vi "PowderDeposition.vi"(8 "error in (no error)":errorcluster, 9 "Com-in":refnum<queue>, 10 "Com-out":refnum<queue>) -> (0 "error out":errorcluster)   [LabVIEW 2013, in "PowderDeposition.lvlib"]
doc: "Use this template to build a producer/consumer design pattern with events to produce queue items. Use this design pattern instead of the User Interface Event Handler pattern for user interfaces when you want to execute code asynchronously in response to an event without slowing the user interface responsiveness."
uses:
  PowderDeposition.lvlib
  Sources/Assembly/Motor-selection.ctl
  Sources/Action/Motor-actions.ctl
  Sources/Main/Options.ctl
  SA-SLMAPI/Sources/Message.lvclass
  Sources/Main/Motor-status.ctl
  Sources/Main/PD-actions.ctl
  Sources/Main/Enqueue-modes.ctl
  Sources/Main/Client-status.ctl
  Sources/Main/Execution-actions.ctl
  Sources/Main/PD-Main.lvclass/PD-Main.ctl
  Sources/Main/Read Assert safe.vi
  Sources/Main/PD-Main.lvclass
  Sources/Assembly/Motor-assembly.lvclass
  Sources/Action/Action.lvclass
panel:
  in  "Clear sequences":bool
  in  "Save sequences":bool
  in  "Load sequences":bool
  in  "Edit action":bool
  in  "Remove from sequence":bool
  in  "Add to sequence":bool
  in  "Available-actions":T1=enum."Move - Relative" caption="Action"
  in  "Execute sequence":bool
  in  "Execute action":bool
  in  "Quick stop":bool
  in  "Toggle help":bool
  out "Motors-status":T2 caption="Status"
  in  "Options":T3
  in  "Activate all":bool
  in  "De-activate all":bool
  in  "Motors-selection":T4 caption="Select motors"
  in  "Motor tabs":T5(tab)
  in  "M1-sequence":i32(listbox) caption="M1 - Action sequence"
  in  "M2-sequence":i32(listbox) caption="M2 - Action sequence"
  in  "M3-sequence":i32(listbox) caption="M3 - Action sequence"
  in  "M4-sequence":i32(listbox) caption="M4 - Action sequence"
  out "Log":string[][](table)
  out "Status":string caption="Status:"
  out "Action:":T6
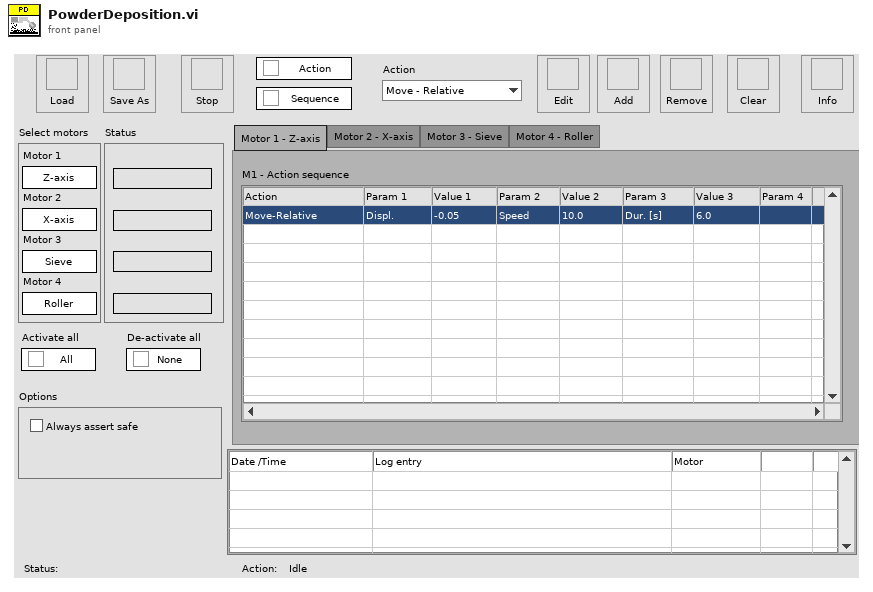
[diagram p1: front panel]
types:
  T1 = typedef "PowderDeposition.lvlib/Action.lvclass/Motor-actions.ctl" = enum16{"Move - Absolute", "Move - Relative", "Move - Timer", "Wait", "Home", "Substrate", "Sieve", "Stop"}
  T2 = typedef "PowderDeposition.lvlib/PD-Main.lvclass/Motor-status.ctl" = cluster{"Motor 1 status":string, "Motor 2 status":string, "Motor 3 status":string, "Motor 4 status":string}
  T3 = typedef "PowderDeposition.lvlib/PD-Main.lvclass/Options.ctl" = cluster{"Assert safe":bool}
  T4 = typedef "PowderDeposition.lvlib/Motor-assembly.lvclass/Motor-selection.ctl" = cluster{"Motor 1":bool, "Motor 2":bool, "Motor 3":bool, "Motor 4":bool}
  T5 = enum32{"Motor 1 - Z-axis", "Motor 2 - X-axis", "Motor 3 - Sieve", "Motor 4 - Roller"}
  T6 = typedef "PowderDeposition.lvlib/PD-Main.lvclass/PD-actions.ctl" = enum16{"Idle", "Initialize", "Signal initialized", "Activate all motors", "Deactivate all motors", "Update motor activity", "Update selected motor", "Update motor status", "Update selected sequence", "Load sequences with dialog", "Load sequences from file", "Save sequences", "Add to sequence", "Remove from sequence", "Clear sequences", "Update available actions", "Create action", "Edit action", "Execute action", "Execute sequences", "Execute seq with assert", "Abort", "Exit"}
  T7 = typedef "PowderDeposition.lvlib/PD-Main.lvclass/Object-reference.ctl" = refnum<data-value>
  T8 = typedef "PowderDeposition.lvlib/PD-Main.lvclass/Client-status.ctl" = enum16{"Idle", "Initialized", "Configured", "Activated", "Started", "Paused", "Stopped", "Reset", "Error", "Exited"}
  T9 = typedef "PowderDeposition.lvlib/PD-Main.lvclass/Execution-actions.ctl" = enum16{"Idle", "Execute action", "Execute sequence", "Execute seq with assert", "Exit"}
  T10 = typedef "PowderDeposition.lvlib/PD-Main.lvclass/Enqueue-modes.ctl" = enum16{"Default", "Priority", "Flush"}
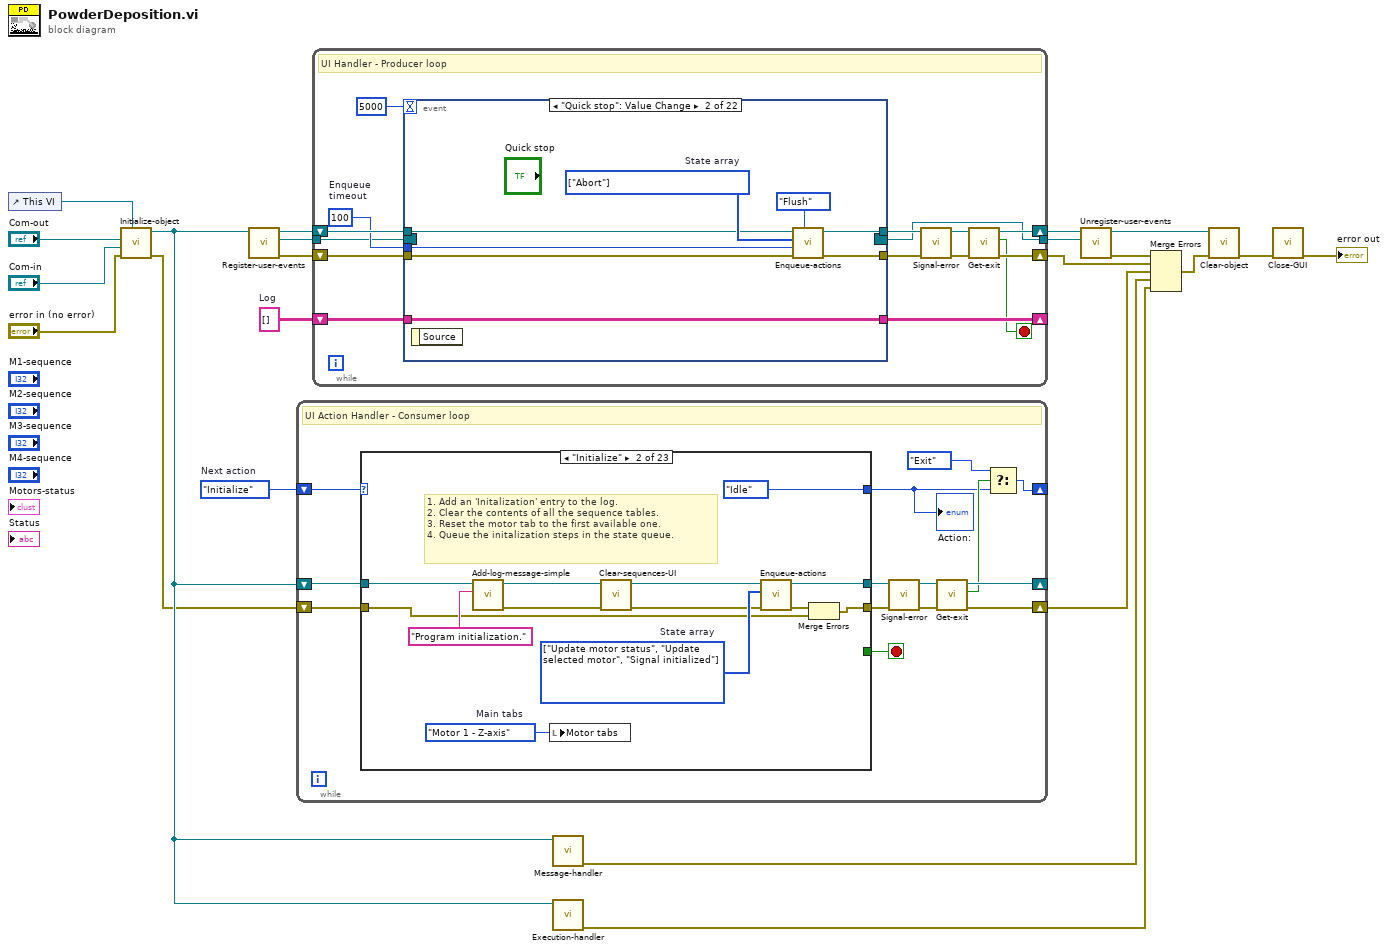
[diagram p0: block diagram]
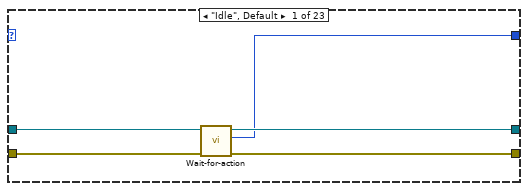
[diagram p2: hidden frame]
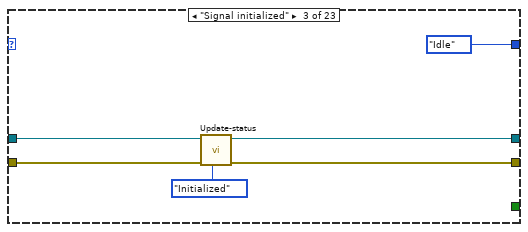
[diagram p3: hidden frame]
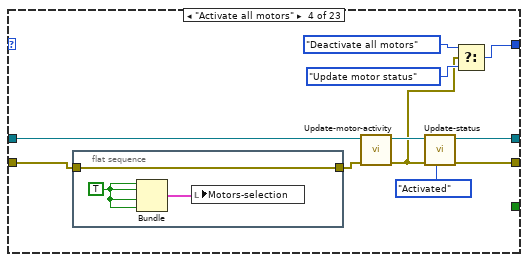
[diagram p4: hidden frame]
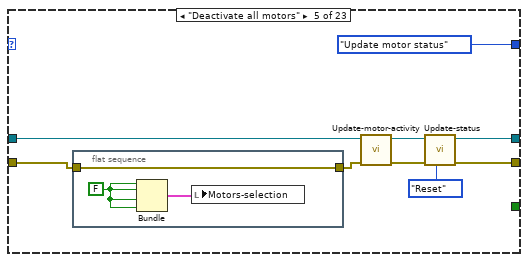
[diagram p5: hidden frame]
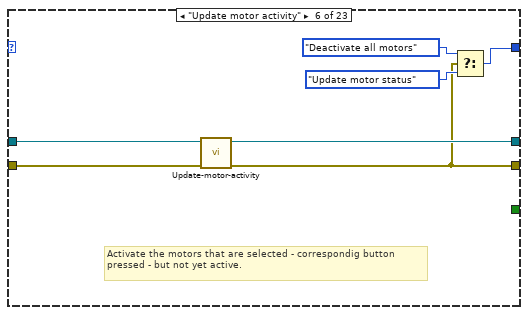
[diagram p6: hidden frame]
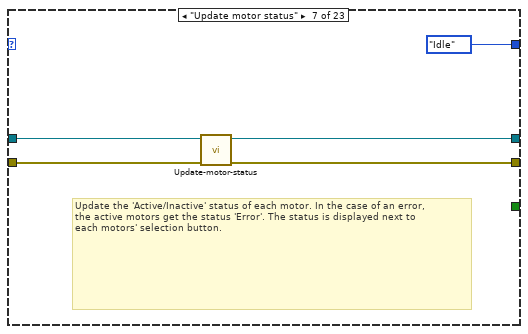
[diagram p7: hidden frame]
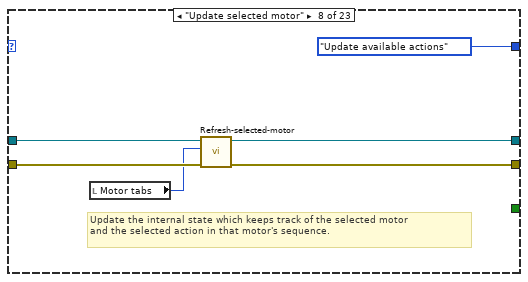
[diagram p8: hidden frame]
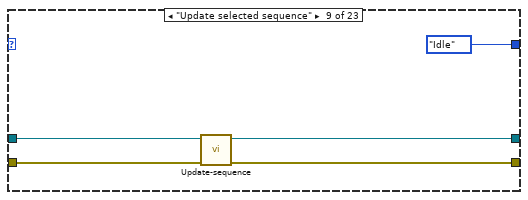
[diagram p9: hidden frame]
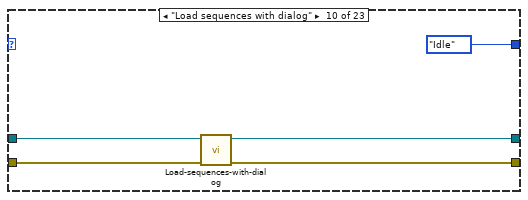
[diagram p10: hidden frame]
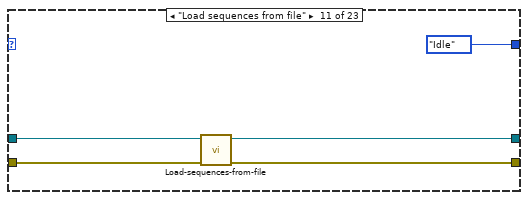
[diagram p11: hidden frame]
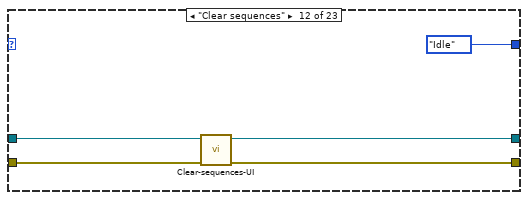
[diagram p12: hidden frame]
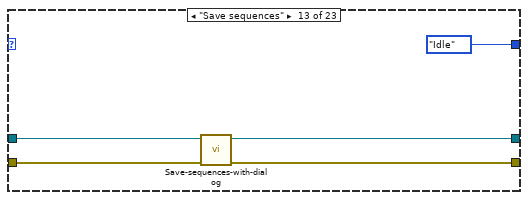
[diagram p13: hidden frame]
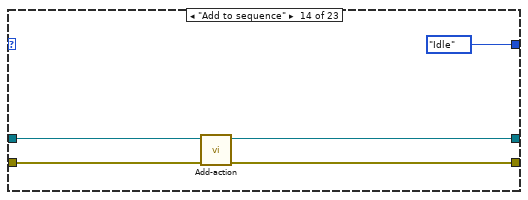
[diagram p14: hidden frame]
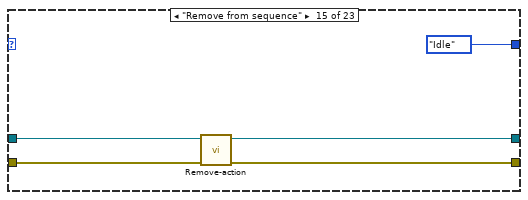
[diagram p15: hidden frame]
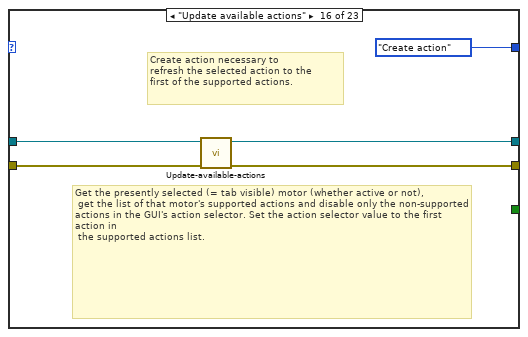
[diagram p16: hidden frame]
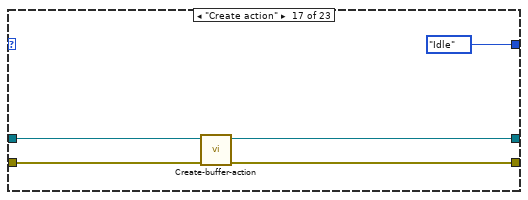
[diagram p17: hidden frame]
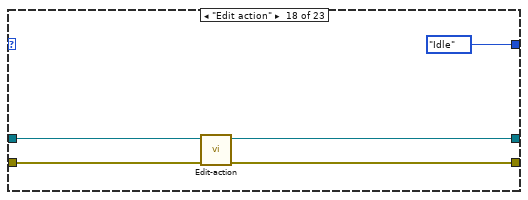
[diagram p18: hidden frame]
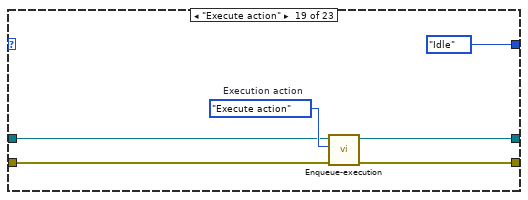
[diagram p19: hidden frame]
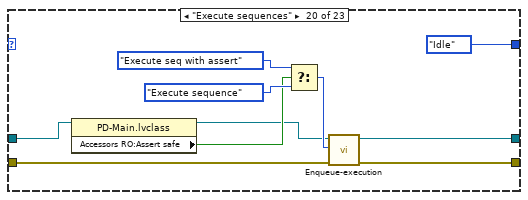
[diagram p20: hidden frame]
diagram:
  w20 = string[][] []  # Log
  w22 = PD-actions."Initialize"  # Next action
  n1 = control-ref of="This VI"() -> (w17:refnum<vi>)
  n2 = call "Initialize-object.vi"("Main VI ref"=w17, "error in (no error)"="error in (no error)", "Client channel"="Com-in", "Server channel"="Com-out") -> ("error out"=w4:errorcluster, "Object ref out"=w7:T7)  [unwired: 6 in]
  n3 = call "Register-user-events.vi"("Object ref in"=w7) -> ("error out"=w14:errorcluster, "Event registration"=w15:refnum<event-registration>, "Object ref out"=w16:T7)  [unwired: 8 in]
  n4 = while {
    shift-right: [w27] -> _
    shift-left: w22 -> [w35]
    shift-right: [w25] -> w21
    shift-left: w4 -> [w34]
    shift-right: [w30] -> _
    shift-left: w7 -> [w33]
    stop <- w36 stop-if-true
    # "UI Action Handler - Consumer loop"
    n5 = case shown="\"Initialize\"" w35 {
      tunnel: [_ _ _ _ _ _ _ _ _ _ _ _ _ _ _ _ _ _ _ _ _ _ TRUE] -> w36
      tunnel: w34 -> [w37 w44 w57 w69 w80 w92 w96 w100 w107 w112 w117 w122 w127 w132 w137 w143 w148 w152 w157 w161 w173 w179 w184]
      tunnel: [w39 w42 w56 w66 w76 w87 w95 w101 w105 w110 w115 w120 w125 w131 w135 w142 w145 w151 w156 w166 w175 w177 w187] -> w24
      tunnel: [w38 PD-actions."Idle" ("Action Handler states") PD-actions."Idle" ("Action Handler states") w62 PD-actions."Update motor status" ("Action Handler states") w88 PD-actions."Idle" ("Action Handler states") PD-actions."Update available actions" ("Action Handler states") PD-actions."Idle" ("Action Handler states") PD-actions."Idle" ("Action Handler states") PD-actions."Idle" ("Action Handler states") PD-actions."Idle" ("Action Handler states") PD-actions."Idle" ("Action Handler states") PD-actions."Idle" ("Action Handler states") PD-actions."Idle" ("Action Handler states") PD-actions."Create action" ("Action Handler states") PD-actions."Idle" ("Action Handler states") PD-actions."Idle" ("Action Handler states") PD-actions."Idle" ("Action Handler states") PD-actions."Idle" ("Action Handler states") PD-actions."Idle" ("Action Handler states") PD-actions."Idle" ("Action Handler states") PD-actions."Exit" ("Action Handler states")] -> w23
      tunnel: w33 -> [w41 w45 w58 w71 w82 w93 w97 w103 w108 w113 w118 w123 w128 w133 w138 w141 w147 w153 w158 w165 w172 w180 w186]
      tunnel: [w40 w51 w55 w65 w77 w91 w94 w102 w106 w111 w116 w121 w126 w130 w136 w140 w146 w150 w155 w163 w174 w178 w188] -> w32
      frame "Idle", Default {
        n6 = call "Wait-for-action.vi"("error in (no error)"=w37, "Object ref in"=w41) -> ("error out"=w39:errorcluster, "Next action"=w38:T6, "Object ref out"=w40:T7)  [unwired: 7 in]
      }
      frame "Initialize" {
        w48 = T5."Motor 1 - Z-axis"  # Main tabs
        w54 = T6[] [enum."Update motor status", enum."Update selected motor", enum."Signal initialized"] items=["Idle", "Initialize", "Signal initialized", "Activate all motors", "Deactivate all motors", "Update motor activity", "Update selected motor", "Update motor status", "Update selected sequence", "Load sequences with dialog", "Load sequences from file", "Save sequences", "Add to sequence", "Remove from sequence", "Clear sequences", "Update available actions", "Create action", "Edit action", "Execute action", "Execute sequences", "Execute seq with assert", "Abort", "Exit"]  # State array
        # "1. Add an 'Initalization' entry to the log.\n2. Clear the contents of all the sequence tables.\n3. Reset the motor tab to the first available one.\n4. Queue the initalization steps in the state queue."
        n7 = call "Add-log-message-simple.vi"("Message"="Program initialization." ("Log message"), "UI in"=w45) -> ("error out"=w49:errorcluster, "UI out"=w50:T7)  [unwired: 8 in]
        n8 = local write "Motor tabs"(w48) -> ()
        n9 = call "Clear-sequences-UI.vi"("error in (no error)"=w49, "Object ref in"=w50) -> ("error out"=w47:errorcluster, "Object ref out"=w46:T7)  [unwired: 8 in]
        n10 = call "Enqueue-actions.vi"("error in (no error)"=w47, "State array"=w54, "State queue in"=w46) -> ("error out"=w43:errorcluster, "State queue out"=w51:T7)  [unwired: 6 in, 1 out]
        n11 = Merge Errors(w43, w44) -> (w42:errorcluster)
      }
      frame "Signal initialized" {
        n12 = call "Update-status.vi"("Status"=Client-status."Initialized", "error in (no error)"=w57, "Object ref in"=w58) -> ("error out"=w56:errorcluster, "Object ref out"=w55:T7)  [unwired: 7 in]
      }
      frame "Activate all motors" {
        n13 = flat-sequence {
          tunnel: w69 -> [w72]
          tunnel: [w72] -> w70
          frame #0 {
            w73 = TRUE
            n14 = Bundle(w73, w73, w73, w73) -> (w74:cluster{bool, bool, bool, bool})  [unwired: 1 in]
            n15 = local write "Motors-selection"(w74) -> ()
          }
        }
        n16 = call "Update-motor-activity.vi"("error in (no error)"=w70, "Data in"=w71) -> ("error out"=w61:errorcluster, "Data out"=w67:T7)  [unwired: 8 in]
        n17 = call "Update-status.vi"("Status"=Client-status."Activated", "error in (no error)"=w61, "Object ref in"=w67) -> ("error out"=w66:errorcluster, "Object ref out"=w65:T7)  [unwired: 7 in]
        n18 = Select(t=PD-actions."Deactivate all motors" ("Action Handler states"), s=w61, f=PD-actions."Update motor status" ("Action Handler states")) -> (s? t:f=w62:T6)
      }
      frame "Deactivate all motors" {
        n19 = flat-sequence {
          tunnel: w80 -> [w84]
          tunnel: [w84] -> w81
          frame #0 {
            w85 = FALSE
            n20 = Bundle(w85, w85, w85, w85) -> (w86:cluster{bool, bool, bool, bool})  [unwired: 1 in]
            n21 = local write "Motors-selection"(w86) -> ()
          }
        }
        n22 = call "Update-motor-activity.vi"("error in (no error)"=w81, "Data in"=w82) -> ("error out"=w75:errorcluster, "Data out"=w78:T7)  [unwired: 8 in]
        n23 = call "Update-status.vi"("Status"=Client-status."Reset", "error in (no error)"=w75, "Object ref in"=w78) -> ("error out"=w76:errorcluster, "Object ref out"=w77:T7)  [unwired: 7 in]
      }
      frame "Update motor activity" {
        # "Activate the motors that are selected - correspondig button pressed - but not yet active."
        n24 = call "Update-motor-activity.vi"("error in (no error)"=w92, "Data in"=w93) -> ("error out"=w87:errorcluster, "Data out"=w91:T7)  [unwired: 8 in]
        n25 = Select(t=PD-actions."Deactivate all motors" ("Action Handler states"), s=w87, f=PD-actions."Update motor status" ("Action Handler states")) -> (s? t:f=w88:T6)
      }
      frame "Update motor status" {
        # "Update the 'Active/Inactive' status of each motor. In the case of an error,\nthe active motors get the status 'Error'. The status is displayed next to \neach motors' selection button."
        n26 = call "Update-motor-status.vi"("error in (no error)"=w96, "Object ref in"=w97) -> ("error out"=w95:errorcluster, "Object ref out"=w94:T7)  [unwired: 8 in]
      }
      frame "Update selected motor" {
        # "Update the internal state which keeps track of the selected motor\nand the selected action in that motor's sequence."
        n27 = local read "Motor tabs"() -> (w99:T5)
        n28 = call "Refresh-selected-motor.vi"("error in (no error)"=w100, "Motor index"=w99, "Object ref in"=w103) -> ("error out"=w101:errorcluster, "Object ref out"=w102:T7)  [unwired: 7 in]
      }
      frame "Update selected sequence" {
        n29 = call "Update-sequence.vi"("error in (no error)"=w107, "Object ref in"=w108) -> ("error out"=w105:errorcluster, "Object ref out"=w106:T7)  [unwired: 8 in]
      }
      frame "Load sequences with dialog" {
        n30 = call "Load-sequences-with-dialog.vi"("error in (no error)"=w112, "Object ref in"=w113) -> ("error out"=w110:errorcluster, "Object ref out"=w111:T7)  [unwired: 8 in]
      }
      frame "Load sequences from file" {
        n31 = call "Load-sequences-from-file.vi"("error in (no error)"=w117, "Object ref in"=w118) -> ("error out"=w115:errorcluster, "Object ref out"=w116:T7)  [unwired: 8 in]
      }
      frame "Clear sequences" {
        n32 = call "Clear-sequences-UI.vi"("error in (no error)"=w122, "Object ref in"=w123) -> ("error out"=w120:errorcluster, "Object ref out"=w121:T7)  [unwired: 8 in]
      }
      frame "Save sequences" {
        n33 = call "Save-sequences-with-dialog.vi"("error in (no error)"=w127, "Object ref in"=w128) -> ("error out"=w125:errorcluster, "Object ref out"=w126:T7)  [unwired: 8 in]
      }
      frame "Add to sequence" {
        n34 = call "Add-action.vi"("error in (no error)"=w132, "Object ref in"=w133) -> ("error out"=w131:errorcluster, "Object ref out"=w130:T7)  [unwired: 8 in]
      }
      frame "Remove from sequence" {
        n35 = call "Remove-action.vi"("error in (no error)"=w137, "Object ref in"=w138) -> ("error out"=w135:errorcluster, "Object ref out"=w136:T7)  [unwired: 8 in]
      }
      frame "Update available actions" {
        # "Get the presently selected (= tab visible) motor (whether active or not),\n get the list of that motor's supported actions and disable only the non-supported\nactions in the GUI's action selector. Set the action selector value to the first action in\n the supported actions list."
        # "Create action necessary to \nrefresh the selected action to the\nfirst of the supported actions."
        n36 = call "Update-available-actions.vi"("error in (no error)"=w143, "Object ref in"=w141) -> ("error out"=w142:errorcluster, "Object ref out"=w140:T7)  [unwired: 8 in]
      }
      frame "Create action" {
        n37 = call "Create-buffer-action.vi"("error in (no error)"=w148, "Object ref in"=w147) -> ("error out"=w145:errorcluster, "Object ref out"=w146:T7)  [unwired: 8 in]
      }
      frame "Edit action" {
        n38 = call "Edit-action.vi"("error in (no error)"=w152, "Object ref in"=w153) -> ("error out"=w151:errorcluster, "Object ref out"=w150:T7)  [unwired: 8 in]
      }
      frame "Execute action" {
        w159 = Execution-actions."Execute action"  # Execution action
        n39 = call "Enqueue-execution.vi"("error in (no error)"=w157, "Execution action"=w159, "State queue in"=w158) -> ("error out"=w156:errorcluster, "State queue out"=w155:T7)  [unwired: 6 in, 1 out]
      }
      frame "Execute sequences" {
        n40 = property class="PD-Main.lvclass"(reference=w165) -> (reference out=w162:T7, "Accessors RO:Assert safe"=w164:bool)  [unwired: 1 in, 1 out]
        n41 = Select(t=Execution-actions."Execute seq with assert" ("Execution action"), s=w164, f=Execution-actions."Execute sequence" ("Execution action")) -> (s? t:f=w167:T9)
        n42 = call "Enqueue-execution.vi"("error in (no error)"=w161, "Execution action"=w167, "State queue in"=w162) -> ("error out"=w166:errorcluster, "State queue out"=w163:T7)  [unwired: 6 in, 1 out]
      }
      frame "Execute seq with assert" {
        n43 = call "Enqueue-execution.vi"("error in (no error)"=w173, "Execution action"=Execution-actions."Execute seq with assert", "State queue in"=w172) -> ("error out"=w175:errorcluster, "State queue out"=w174:T7)  [unwired: 6 in, 1 out]
      }
      frame "Abort" {
        n44 = call "Abort.vi"("error in (no error)"=w179, "Object ref in"=w180) -> ("error out"=w177:errorcluster, "Object ref out"=w178:T7)  [unwired: 8 in]
      }
      frame "Exit" {
        w193 = Execution-actions."Exit"  # Execution action
        w182 = TRUE  # Exit
        n45 = call "Set-abort.vi"("error in (no error)"=w184, "Abort"=w182, "Object ref in"=w186) -> ("error out"=w183:errorcluster, "Object ref out"=w185:T7)  [unwired: 7 in]
        n46 = call "Set-exit.vi"("error in (no error)"=w183, "Exit"=w182, "Object ref in"=w185) -> ("error out"=w191:errorcluster, "Object ref out"=w192:T7)  [unwired: 7 in]
        n47 = call "Enqueue-execution.vi"("error in (no error)"=w191, "Execution action"=w193, "State queue in"=w192) -> ("error out"=w189:errorcluster, "State queue out"=w190:T7)  [unwired: 6 in, 1 out]
        n48 = call "Trigger-message-handler.vi"("error in (no error)"=w189, "Object ref in"=w190) -> ("error out"=w187:errorcluster, "Object ref out"=w188:T7)  [unwired: 8 in]
      }
    }
    "Action:" <- w23
    n49 = call "Signal-error.vi"("error in (no error)"=w24, "Data in"=w32) -> ("error out"=w29:errorcluster, "Data out"=w31:T7)  [unwired: 8 in]
    n50 = call "Get-exit.vi"("error in (no error)"=w29, "Object ref in"=w31) -> ("error out"=w25:errorcluster, "Exit?"=w28:bool, "Object ref out"=w30:T7)  [unwired: 7 in]
    n51 = Select(t=PD-actions."Exit", s=w28, f=w23) -> (s? t:f=w27:T6)
  }
  n52 = while {
    shift-right: [w200] -> w3
    shift-left: w14 -> [w209]
    tunnel: w15 -> [w206]
    tunnel: [w196] -> w12
    shift-right: [w204] -> _
    shift-left: w20 -> [w205]
    shift-right: [w203] -> w13
    shift-left: w16 -> [w210]
    stop <- w197 stop-if-true
    w207 = 100  # Enqueue timeout
    # "UI Handler - Producer loop"
    n53 = event shown="[1] \"Quick stop\": Value Change" {
      selector: w206 -> [_ _ _ _ _ _ _ _ _ _ _ _ _ _ _ _ _ _ _ _ _ _]
      dyn-events: [_ _ _ _ _ _ _ _ _ _ _ _ _ _ _ _ _ _ _ _ _ _] -> w196
      timeout: 5000 -> [_ _ _ _ _ _ _ _ _ _ _ _ _ _ _ _ _ _ _ _ _ _]
      tunnel: w210 -> [w211 w218 w225 w231 w238 w245 w252 w258 w265 w272 w279 w286 w293 w299 w306 w315 w322 w329 w334 w344 w348 w357]
      tunnel: w209 -> [w212 w219 w226 w232 w239 w246 w253 w260 w267 w274 w281 w288 w295 w300 w307 w312 w320 w326 w336 w343 w352 w355]
      tunnel: [w212 w220 w223 w233 w240 w247 w254 w261 w268 w275 w282 w289 w296 w301 w308 w317 w324 w331 w336 w341 w352 w353] -> w198
      tunnel: w207 -> [_ w217 _ w230 w237 w244 w251 w259 w266 w273 w280 w287 w294 w298 w305 w316 w323 w330 _ _ _ _]
      tunnel: w205 -> [w213 w215 w227 w229 w236 w243 w250 w257 w264 w271 w278 w285 w292 w304 w311 w314 w321 w328 w335 w346 w351 w363]
      tunnel: [w213 w215 w227 w229 w236 w243 w250 w257 w264 w271 w278 w285 w292 w304 w311 w314 w321 w328 w335 w346 w350 w363] -> w204
      tunnel: [w211 w214 w224 w228 w235 w242 w249 w256 w263 w270 w277 w284 w291 w302 w309 w313 w319 w327 w334 w342 w348 w354] -> w202
      event Timeout {
        n54 = event-data() -> ()  [unwired: 1 in, 1 out]
      }
      event "Quick stop": Value Change {
        w221 = T6[] [enum."Abort"] items=["Idle", "Initialize", "Signal initialized", "Activate all motors", "Deactivate all motors", "Update motor activity", "Update selected motor", "Update motor status", "Update selected sequence", "Load sequences with dialog", "Load sequences from file", "Save sequences", "Add to sequence", "Remove from sequence", "Clear sequences", "Update available actions", "Create action", "Edit action", "Execute action", "Execute sequences", "Execute seq with assert", "Abort", "Exit"]  # State array
        n55 = event-data() -> ()  [unwired: 1 in, 1 out]
        n56 = call "Enqueue-actions.vi"("Enqueue mode"=Enqueue-modes."Flush", "error in (no error)"=w219, "Timeout (ms)"=w217, "State array"=w221, "State queue in"=w218) -> ("error out"=w220:errorcluster, "State queue out"=w214:T7)  [unwired: 4 in, 1 out]
      }
      event Value Change {
        n57 = event-data() -> ()  [unwired: 1 in, 1 out]
        n58 = call "Set-options.vi"("error in (no error)"=w226, "Options"="Options", "Object ref in"=w225) -> ("error out"=w223:errorcluster, "Object ref out"=w224:T7)  [unwired: 7 in]
      }
      event "Edit action": Value Change {
        w234 = T6[] [enum."Edit action"] items=["Idle", "Initialize", "Signal initialized", "Activate all motors", "Deactivate all motors", "Update motor activity", "Update selected motor", "Update motor status", "Update selected sequence", "Load sequences with dialog", "Load sequences from file", "Save sequences", "Add to sequence", "Remove from sequence", "Clear sequences", "Update available actions", "Create action", "Edit action", "Execute action", "Execute sequences", "Execute seq with assert", "Abort", "Exit"]  # State array
        n59 = event-data() -> ()  [unwired: 1 in, 1 out]
        n60 = call "Enqueue-actions.vi"("error in (no error)"=w232, "Timeout (ms)"=w230, "State array"=w234, "State queue in"=w231) -> ("error out"=w233:errorcluster, "State queue out"=w228:T7)  [unwired: 5 in, 1 out]
      }
      event "Save sequences": Value Change {
        w241 = T6[] [enum."Save sequences"] items=["Idle", "Initialize", "Signal initialized", "Activate all motors", "Deactivate all motors", "Update motor activity", "Update selected motor", "Update motor status", "Update selected sequence", "Load sequences with dialog", "Load sequences from file", "Save sequences", "Add to sequence", "Remove from sequence", "Clear sequences", "Update available actions", "Create action", "Edit action", "Execute action", "Execute sequences", "Execute seq with assert", "Abort", "Exit"]  # State array
        n61 = event-data() -> ()  [unwired: 1 in, 1 out]
        n62 = call "Enqueue-actions.vi"("error in (no error)"=w239, "Timeout (ms)"=w237, "State array"=w241, "State queue in"=w238) -> ("error out"=w240:errorcluster, "State queue out"=w235:T7)  [unwired: 5 in, 1 out]
      }
      event "Load sequences": Value Change {
        w248 = T6[] [enum."Load sequences with dialog"] items=["Idle", "Initialize", "Signal initialized", "Activate all motors", "Deactivate all motors", "Update motor activity", "Update selected motor", "Update motor status", "Update selected sequence", "Load sequences with dialog", "Load sequences from file", "Save sequences", "Add to sequence", "Remove from sequence", "Clear sequences", "Update available actions", "Create action", "Edit action", "Execute action", "Execute sequences", "Execute seq with assert", "Abort", "Exit"]  # State array
        n63 = event-data() -> ()  [unwired: 1 in, 1 out]
        n64 = call "Enqueue-actions.vi"("error in (no error)"=w246, "Timeout (ms)"=w244, "State array"=w248, "State queue in"=w245) -> ("error out"=w247:errorcluster, "State queue out"=w242:T7)  [unwired: 5 in, 1 out]
      }
      event "Clear sequences": Value Change {
        w255 = T6[] [enum."Clear sequences"] items=["Idle", "Initialize", "Signal initialized", "Activate all motors", "Deactivate all motors", "Update motor activity", "Update selected motor", "Update motor status", "Update selected sequence", "Load sequences with dialog", "Load sequences from file", "Save sequences", "Add to sequence", "Remove from sequence", "Clear sequences", "Update available actions", "Create action", "Edit action", "Execute action", "Execute sequences", "Execute seq with assert", "Abort", "Exit"]  # State array
        n65 = event-data() -> ()  [unwired: 1 in, 1 out]
        n66 = call "Enqueue-actions.vi"("error in (no error)"=w253, "Timeout (ms)"=w251, "State array"=w255, "State queue in"=w252) -> ("error out"=w254:errorcluster, "State queue out"=w249:T7)  [unwired: 5 in, 1 out]
      }
      event "Remove from sequence": Value Change {
        w262 = T6[] [enum."Remove from sequence"] items=["Idle", "Initialize", "Signal initialized", "Activate all motors", "Deactivate all motors", "Update motor activity", "Update selected motor", "Update motor status", "Update selected sequence", "Load sequences with dialog", "Load sequences from file", "Save sequences", "Add to sequence", "Remove from sequence", "Clear sequences", "Update available actions", "Create action", "Edit action", "Execute action", "Execute sequences", "Execute seq with assert", "Abort", "Exit"]  # State array
        n67 = event-data() -> ()  [unwired: 1 in, 1 out]
        n68 = call "Enqueue-actions.vi"("error in (no error)"=w260, "Timeout (ms)"=w259, "State array"=w262, "State queue in"=w258) -> ("error out"=w261:errorcluster, "State queue out"=w256:T7)  [unwired: 5 in, 1 out]
      }
      event "Motor tabs": Value Change {
        w269 = T6[] [enum."Update selected motor", enum."Update selected sequence"] items=["Idle", "Initialize", "Signal initialized", "Activate all motors", "Deactivate all motors", "Update motor activity", "Update selected motor", "Update motor status", "Update selected sequence", "Load sequences with dialog", "Load sequences from file", "Save sequences", "Add to sequence", "Remove from sequence", "Clear sequences", "Update available actions", "Create action", "Edit action", "Execute action", "Execute sequences", "Execute seq with assert", "Abort", "Exit"]  # State array
        n69 = event-data() -> ()  [unwired: 1 in, 1 out]
        n70 = call "Enqueue-actions.vi"("error in (no error)"=w267, "Timeout (ms)"=w266, "State array"=w269, "State queue in"=w265) -> ("error out"=w268:errorcluster, "State queue out"=w263:T7)  [unwired: 5 in, 1 out]
      }
      event "M1-sequence", "M2-sequence", "M3-sequence", "M4-sequence": Mouse Up {
        w276 = T6[] [enum."Update selected motor"] items=["Idle", "Initialize", "Signal initialized", "Activate all motors", "Deactivate all motors", "Update motor activity", "Update selected motor", "Update motor status", "Update selected sequence", "Load sequences with dialog", "Load sequences from file", "Save sequences", "Add to sequence", "Remove from sequence", "Clear sequences", "Update available actions", "Create action", "Edit action", "Execute action", "Execute sequences", "Execute seq with assert", "Abort", "Exit"]  # State array
        n71 = event-data() -> ()  [unwired: 1 in, 1 out]
        n72 = call "Enqueue-actions.vi"("error in (no error)"=w274, "Timeout (ms)"=w273, "State array"=w276, "State queue in"=w272) -> ("error out"=w275:errorcluster, "State queue out"=w270:T7)  [unwired: 5 in, 1 out]
      }
      event "M1-sequence", "M2-sequence", "M3-sequence", "M4-sequence": Double Click {
        w283 = T6[] [enum."Update selected motor", enum."Edit action"] items=["Idle", "Initialize", "Signal initialized", "Activate all motors", "Deactivate all motors", "Update motor activity", "Update selected motor", "Update motor status", "Update selected sequence", "Load sequences with dialog", "Load sequences from file", "Save sequences", "Add to sequence", "Remove from sequence", "Clear sequences", "Update available actions", "Create action", "Edit action", "Execute action", "Execute sequences", "Execute seq with assert", "Abort", "Exit"]  # State array
        n73 = event-data() -> ()  [unwired: 1 in, 1 out]
        n74 = call "Enqueue-actions.vi"("error in (no error)"=w281, "Timeout (ms)"=w280, "State array"=w283, "State queue in"=w279) -> ("error out"=w282:errorcluster, "State queue out"=w277:T7)  [unwired: 5 in, 1 out]
      }
      event "Add to sequence": Value Change {
        w290 = T6[] [enum."Add to sequence"] items=["Idle", "Initialize", "Signal initialized", "Activate all motors", "Deactivate all motors", "Update motor activity", "Update selected motor", "Update motor status", "Update selected sequence", "Load sequences with dialog", "Load sequences from file", "Save sequences", "Add to sequence", "Remove from sequence", "Clear sequences", "Update available actions", "Create action", "Edit action", "Execute action", "Execute sequences", "Execute seq with assert", "Abort", "Exit"]  # State array
        n75 = event-data() -> ()  [unwired: 1 in, 1 out]
        n76 = call "Enqueue-actions.vi"("error in (no error)"=w288, "Timeout (ms)"=w287, "State array"=w290, "State queue in"=w286) -> ("error out"=w289:errorcluster, "State queue out"=w284:T7)  [unwired: 5 in, 1 out]
      }
      event Value Change {
        w297 = T6[] [enum."Create action"] items=["Idle", "Initialize", "Signal initialized", "Activate all motors", "Deactivate all motors", "Update motor activity", "Update selected motor", "Update motor status", "Update selected sequence", "Load sequences with dialog", "Load sequences from file", "Save sequences", "Add to sequence", "Remove from sequence", "Clear sequences", "Update available actions", "Create action", "Edit action", "Execute action", "Execute sequences", "Execute seq with assert", "Abort", "Exit"]  # State array
        n77 = event-data() -> ()  [unwired: 1 in, 1 out]
        n78 = call "Enqueue-actions.vi"("error in (no error)"=w295, "Timeout (ms)"=w294, "State array"=w297, "State queue in"=w293) -> ("error out"=w296:errorcluster, "State queue out"=w291:T7)  [unwired: 5 in, 1 out]
      }
      event "Execute action": Value Change {
        w303 = T6[] [enum."Execute action"] items=["Idle", "Initialize", "Signal initialized", "Activate all motors", "Deactivate all motors", "Update motor activity", "Update selected motor", "Update motor status", "Update selected sequence", "Load sequences with dialog", "Load sequences from file", "Save sequences", "Add to sequence", "Remove from sequence", "Clear sequences", "Update available actions", "Create action", "Edit action", "Execute action", "Execute sequences", "Execute seq with assert", "Abort", "Exit"]  # State array
        n79 = event-data() -> ()  [unwired: 1 in, 1 out]
        n80 = call "Enqueue-actions.vi"("error in (no error)"=w300, "Timeout (ms)"=w298, "State array"=w303, "State queue in"=w299) -> ("error out"=w301:errorcluster, "State queue out"=w302:T7)  [unwired: 5 in, 1 out]
      }
      event "Execute sequence": Value Change {
        w310 = T6[] [enum."Execute sequences"] items=["Idle", "Initialize", "Signal initialized", "Activate all motors", "Deactivate all motors", "Update motor activity", "Update selected motor", "Update motor status", "Update selected sequence", "Load sequences with dialog", "Load sequences from file", "Save sequences", "Add to sequence", "Remove from sequence", "Clear sequences", "Update available actions", "Create action", "Edit action", "Execute action", "Execute sequences", "Execute seq with assert", "Abort", "Exit"]  # State array
        n81 = event-data() -> ()  [unwired: 1 in, 1 out]
        n82 = call "Enqueue-actions.vi"("error in (no error)"=w307, "Timeout (ms)"=w305, "State array"=w310, "State queue in"=w306) -> ("error out"=w308:errorcluster, "State queue out"=w309:T7)  [unwired: 5 in, 1 out]
      }
      event "Activate all": Value Change {
        w318 = T6[] [enum."Activate all motors"] items=["Idle", "Initialize", "Signal initialized", "Activate all motors", "Deactivate all motors", "Update motor activity", "Update selected motor", "Update motor status", "Update selected sequence", "Load sequences with dialog", "Load sequences from file", "Save sequences", "Add to sequence", "Remove from sequence", "Clear sequences", "Update available actions", "Create action", "Edit action", "Execute action", "Execute sequences", "Execute seq with assert", "Abort", "Exit"]  # State array
        n83 = event-data() -> ()  [unwired: 1 in, 1 out]
        n84 = call "Enqueue-actions.vi"("error in (no error)"=w312, "Timeout (ms)"=w316, "State array"=w318, "State queue in"=w315) -> ("error out"=w317:errorcluster, "State queue out"=w313:T7)  [unwired: 5 in, 1 out]
      }
      event Value Change {
        w325 = T6[] [enum."Update motor activity"] items=["Idle", "Initialize", "Signal initialized", "Activate all motors", "Deactivate all motors", "Update motor activity", "Update selected motor", "Update motor status", "Update selected sequence", "Load sequences with dialog", "Load sequences from file", "Save sequences", "Add to sequence", "Remove from sequence", "Clear sequences", "Update available actions", "Create action", "Edit action", "Execute action", "Execute sequences", "Execute seq with assert", "Abort", "Exit"]  # State array
        n85 = event-data() -> ()  [unwired: 1 in, 1 out]
        n86 = call "Enqueue-actions.vi"("error in (no error)"=w320, "Timeout (ms)"=w323, "State array"=w325, "State queue in"=w322) -> ("error out"=w324:errorcluster, "State queue out"=w319:T7)  [unwired: 5 in, 1 out]
      }
      event "De-activate all": Value Change {
        w332 = T6[] [enum."Deactivate all motors"] items=["Idle", "Initialize", "Signal initialized", "Activate all motors", "Deactivate all motors", "Update motor activity", "Update selected motor", "Update motor status", "Update selected sequence", "Load sequences with dialog", "Load sequences from file", "Save sequences", "Add to sequence", "Remove from sequence", "Clear sequences", "Update available actions", "Create action", "Edit action", "Execute action", "Execute sequences", "Execute seq with assert", "Abort", "Exit"]  # State array
        n87 = event-data() -> ()  [unwired: 1 in, 1 out]
        n88 = call "Enqueue-actions.vi"("error in (no error)"=w326, "Timeout (ms)"=w330, "State array"=w332, "State queue in"=w329) -> ("error out"=w331:errorcluster, "State queue out"=w327:T7)  [unwired: 5 in, 1 out]
      }
      event "Toggle help": Value Change {
        n89 = event-data() -> ()  [unwired: 1 in, 1 out]
        n90 = Control Help Window(1:"Toggle help") -> ()  [unwired: 1 in]
      }
      event Panel Close? {
        w340 = T6[] [enum."Exit"] items=["Idle", "Initialize", "Signal initialized", "Activate all motors", "Deactivate all motors", "Update motor activity", "Update selected motor", "Update motor status", "Update selected sequence", "Load sequences with dialog", "Load sequences from file", "Save sequences", "Add to sequence", "Remove from sequence", "Clear sequences", "Update available actions", "Create action", "Edit action", "Execute action", "Execute sequences", "Execute seq with assert", "Abort", "Exit"]  # State array
        w345 = TRUE  # Exit
        w347 = TRUE  # Discard?
        n91 = event-data() -> ()  [unwired: 1 in, 1 out]
        n92 = call "Set-exit.vi"("error in (no error)"=w343, "Exit"=w345, "Object ref in"=w344) -> ("error out"=w337:errorcluster, "Object ref out"=w338:T7)  [unwired: 7 in]
        n93 = call "Enqueue-actions.vi"("Enqueue mode"=Enqueue-modes."Flush", "error in (no error)"=w337, "State array"=w340, "State queue in"=w338) -> ("error out"=w341:errorcluster, "State queue out"=w342:T7)  [unwired: 5 in, 1 out]
        n94 = event-data("Discard?"=w347) -> ()  [unwired: 1 in, 1 out]
      }
      event User Event {
        n95 = event-data() -> ("Log rule"=w349:string[])  [unwired: 1 in]
        n96 = Build Array (concatenate)(w349, w351) -> (w350:string[][])
        "Log" <- w350
      }
      event User Event {
        n97 = event-data() -> ("status"=w362:bool, "code"=w360:i32, "source"=w359:string)  [unwired: 1 in]
        n98 = Bundle By Name(cluster=errorcluster {"status"=FALSE, "code"=0, "source"=""} ("error constant"), "status"=w362, "code"=w360, "source"=w359) -> (w358:errorcluster)
        n99 = Merge Errors(w358, w355) -> (w356:errorcluster)
        n100 = call "Process-error.vi"("error in (no error)"=w356, "Data in"=w357) -> ("error out"=w353:errorcluster, "Data out"=w354:T7)  [unwired: 8 in]
      }
    }
    n101 = call "Signal-error.vi"("error in (no error)"=w198, "Data in"=w202) -> ("error out"=w199:errorcluster, "Data out"=w201:T7)  [unwired: 8 in]
    n102 = call "Get-exit.vi"("error in (no error)"=w199, "Object ref in"=w201) -> ("error out"=w200:errorcluster, "Exit?"=w197:bool, "Object ref out"=w203:T7)  [unwired: 7 in]
  }
  n103 = call "Message-handler.vi"("PD in"=w7) -> ("error out"=w6:errorcluster)  [unwired: 9 in, 1 out]
  n104 = call "Execution-handler.vi"("Object ref in"=w7) -> ("error out"=w5:errorcluster)  [unwired: 9 in, 1 out]
  n105 = call "Unregister-user-events.vi"("Event registration"=w12, "Object ref in"=w13) -> ("error out"=w11:errorcluster, "Object ref out"=w8:T7)  [unwired: 8 in]
  n106 = Merge Errors(w11, w3, w21, w6, w5) -> (w9:errorcluster)
  n107 = call "Clear-object.vi"("error in (no error)"=w9, "Object ref in"=w8) -> ("error out"=w2:errorcluster)  [unwired: 9 in]
  n108 = call "Close-GUI.vi"("error in (no error)"=w2) -> ("error out"=→"error out":errorcluster)  [unwired: 10 in]
